vi "BrainStemExample_LEDToggle.vi"() -> ()   [LabVIEW 2015, in "BrainStem4LabView.lvlib"]
uses:
  BrainStem_DLL_Import/BrainStem4LabView.lvlib
panel:
  out "LED":bool
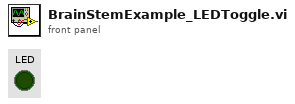
[diagram p1: front panel]
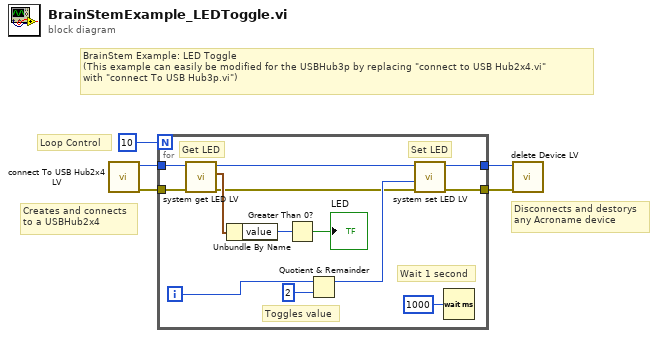
[diagram p0: block diagram]
diagram:
  # "Loop Control"
  # "Disconnects and destorys\nany Acroname device"
  # "Creates and connects\nto a USBHub2x4"
  # "BrainStem Example: LED Toggle\n(This example can easily be modified for the USBHub3p by replacing \"connect to USB Hub2x4.vi\"\nwith \"connect To USB Hub3p.vi\")"
  n1 = call "connect To USB Hub2x4 LV.vi"() -> ("error out"=w2:errorcluster, "id out"=w3:i32)  [unwired: 9 in, 1 out]
  n2 = for {
    N: 10 -> [_]
    tunnel: [w11] -> w4
    tunnel: w3 -> [w14]
    tunnel: w2 -> [w9]
    tunnel: [w7] -> w1
    i -> [w17]
    # "Wait 1 second"
    # "Toggles value"
    # "Set LED"
    # "Get LED"
    n3 = call "system get LED LV.vi"("error in (no error)"=w9, "id"=w14) -> ("error out"=w8:errorcluster, "result out"=w13:cluster{"value":i32, "error":i32}, "id out"=w12:i32)  [unwired: 7 in]
    n4 = Unbundle By Name(w13) -> ("value"=w16:i32)
    n5 = Greater Than 0?(x=w16) -> (x > 0?=→"LED":bool)
    n6 = Quotient & Remainder(x=w17, y=2) -> (x-y*floor(x/y)=w10:i32)  [unwired: 1 out]
    n7 = call "system set LED LV.vi"("error in (no error)"=w8, "LED"=w10, "id"=w12) -> ("error out"=w7:errorcluster, "id out"=w11:i32)  [unwired: 6 in, 1 out]
    n8 = Wait (ms)(milliseconds to wait=1000) -> ()  [unwired: 1 out]
  }
  n9 = call "delete Device LV.vi"("error in (no error)"=w1, "id"=w4) -> ()  [unwired: 8 in, 2 out]
